vi "Get Named Tag.vi"(8 "error in (no error)":errorcluster, 10 "ID":string, 11 "Raw Message in":refnum<class "Raw Message.lvclass">) -> (0 "error out":errorcluster, 2 "Tags":refnum<class "Basic Type.lvclass">[](array[class]), 3 "Raw Message out":refnum<class "Raw Message.lvclass">)   [LabVIEW 2020]
uses:
  Raw Message.lvclass/Raw Message.ctl
  Raw Message.lvclass
  E:/Labview/LV 2020/Libs/LV Protobuf Raw/Source/Tag/Basic Type.lvclass
  E:/Labview/LV 2020/Libs/LV Protobuf Raw/Source/Proto Value/Proto Type.lvclass
  E:/Labview/LV 2020/Libs/LV Protobuf Raw/Source/Type Serializer/Type Serializer.lvclass
  E:/Labview/LV 2020/Libs/LV Protobuf Raw/Source/String Representable/String Representable.lvclass
  E:/Labview/LV 2020/Libs/LV Protobuf Raw/Source/Wire Type Group/Wire Type Group.lvclass
  E:/Labview/LV 2020/Libs/LV Protobuf Raw/Source/LEN Encoder/LEN.lvclass
  E:/Labview/LV 2020/Libs/LV Protobuf Raw/Source/Message/Raw Message.lvclass
  Tag/Basic Type.lvclass
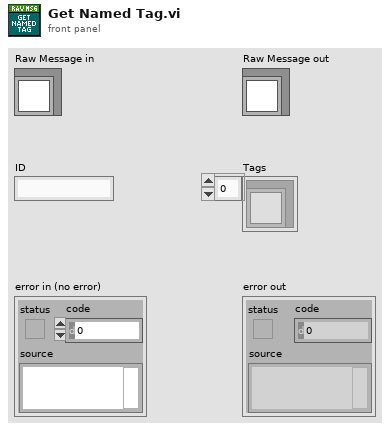
[diagram p1: front panel]
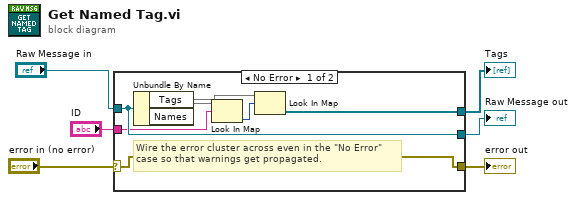
[diagram p0: block diagram]
diagram:
  n1 = case shown="No Error" "error in (no error)" {
    selector: "error in (no error)" -> [w13 w15]
    tunnel: [w13 w15] -> w5
    tunnel: [w12 w14] -> w3
    tunnel: "Raw Message in" -> [w12 w14]
    tunnel: "ID" -> [w8 _]
    tunnel: [w10 _] -> w1
    frame No Error {
      # "Wire the error cluster across even in the \"No Error\"\ncase so that warnings get propagated."
      n2 = Unbundle By Name(w12) -> ("Tags"=w11, "Names"=w9)
      n3 = Look In Map(map=w9, key=w8) -> (value=w7:u32)  [unwired: 1 in, 1 out]
      n4 = Look In Map(map=w11, key=w7) -> (value=w10:refnum<class "Basic Type.lvclass">[])  [unwired: 1 in, 1 out]
    }
    frame Error {
    }
  }
  "error out" <- w5
  "Raw Message out" <- w3
  "Tags" <- w1
